vi "Init.vi"(4 "Telemtry Config (Multicast)":T1, 5 "EventLogger":refnum<class "EventLoggingService.lvclass">, 6 "Bind Address (Any)":string="0.0.0.0", 8 "error in (no error)":errorcluster, 9 "SequenceCountService":refnum<class "SequenceCountService.lvclass">, 10 "ChannelService":refnum<class "ChannelService.lvclass">) -> (0 "error out":errorcluster, 3 "RemoteDataService out":refnum<class "RemoteDataService.lvclass">)   [LabVIEW 2020, in "Vecto.lvlib" / "RemoteDataService.lvclass"]
uses:
  RemoteDataService.lvclass
  ChannelService/ChannelService.lvclass
  SequenceCountService/SequenceCountService.lvclass
  EventLoggingService/EventLoggingService.lvclass
  VectoConfig/Telemetry Config.ctl
  VectoConfig/Telemetry Routing.ctl
  VectoConfig/Endpoint.ctl
  Publish Group Data.ctl
  lv-protoc/LV-Proto/Message/Message.lvclass
  Group Data Type.ctl
  Event Level.ctl
  RemoteDataService.lvclass/RemoteDataService.ctl
  EventLoggingService/EventLoggingService.lvclass/EventLoggingService.ctl
  <vilib>/Utility/error.llb/Error Cluster From Error Code.vi
  EventLogHandler/EventLogHandler.lvclass
  VectoConfig/VectoConfig.lvlib
  Vecto.lvlib
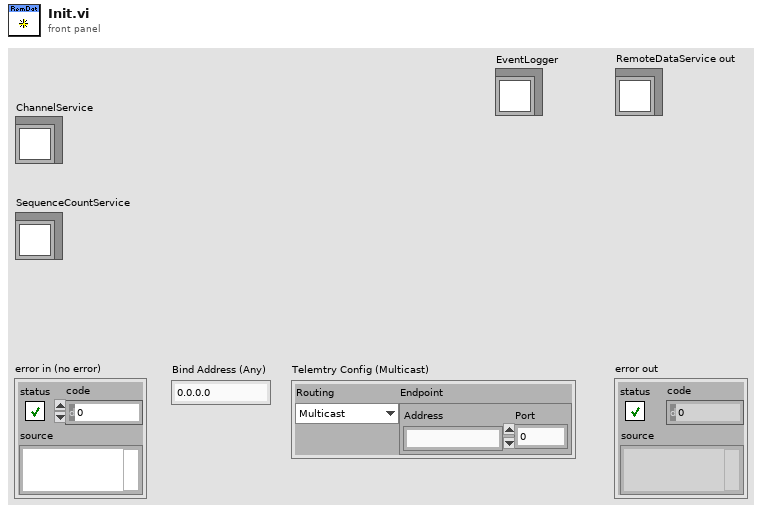
[diagram p1: front panel]
types:
  T1 = typedef "VectoConfig.lvlib/Telemetry Config.ctl" = cluster{"Routing":T2, "Endpoint":T3}
  T2 = typedef "VectoConfig.lvlib/Telemetry Routing.ctl" = enum16{"Multicast", "Unicast"}
  T3 = typedef "VectoConfig.lvlib/Endpoint.ctl" = cluster{"Address":string, "Port":u16}
  T4 = typedef "Vecto.lvlib/Event Level.ctl" = enum16{"Debug", "Info", "Warning", "Error"}
  T5 = typedef "Vecto.lvlib/RemoteDataService.lvclass/Publish Group Data.ctl" = cluster{"Data Msg":refnum<class "Message.lvclass">, "Group Name":string, "Data Type":T6}
  T6 = typedef "VectoConfig.lvlib/Group Data Type.ctl" = enum16{"Double", "String", "Bool"}
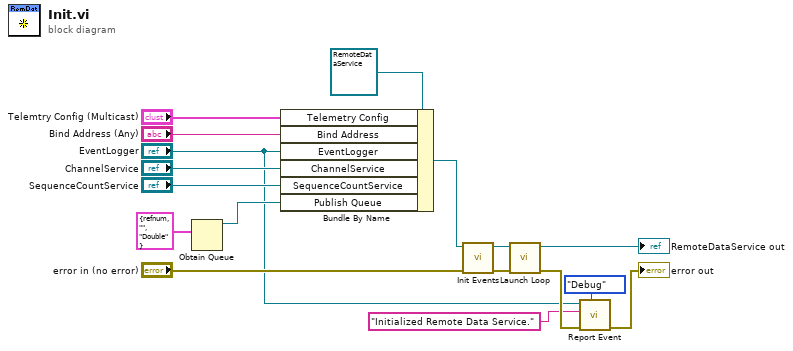
[diagram p0: block diagram]
diagram:
  n1 = Obtain Queue(element data type=T5 {"Data Msg"=refnum, "Group Name"="", "Data Type"=enum."Double"} ("Publish Group Data")) -> (queue out=w8:refnum<queue>)  [unwired: 4 in, 2 out]
  n2 = Bundle By Name(cluster=refnum<class "RemoteDataService.lvclass"> refnum ("RemoteDataService in"), "Telemetry Config"="Telemtry Config (Multicast)", "Bind Address"="Bind Address (Any)", "EventLogger"="EventLogger", "ChannelService"="ChannelService", "SequenceCountService"="SequenceCountService", "Publish Queue"=w8) -> (w13:refnum<class "RemoteDataService.lvclass">)
  n3 = call "Init Events.vi"("error in (no error)"="error in (no error)", "RemoteDataService in"=w13) -> ("error out"=w14:errorcluster, "RemoteDataService out"=w3:refnum<class "RemoteDataService.lvclass">)  [unwired: 8 in]
  n4 = call "Launch Loop.vi"("error in (no error)"=w14, "RemoteDataService in"=w3) -> ("error out"=w11:errorcluster, "RemoteDataService out"=→"RemoteDataService out":refnum<class "RemoteDataService.lvclass">)  [unwired: 8 in]
  n5 = call "Report Event.vi"("Event Level (Info)"=Event_Level."Debug", "error in (no error)"=w11, "Message"="Initialized Remote Data Service.", "EventLoggingService in"="EventLogger") -> ("error out"=→"error out":errorcluster)  [unwired: 6 in, 1 out]
